vi "X_MN_4352.vi"(4 "u":dbl format="%#_13g") -> (1 "y":dbl)   [LabVIEW 2015]
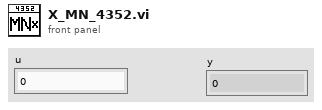
[diagram p1: front panel]
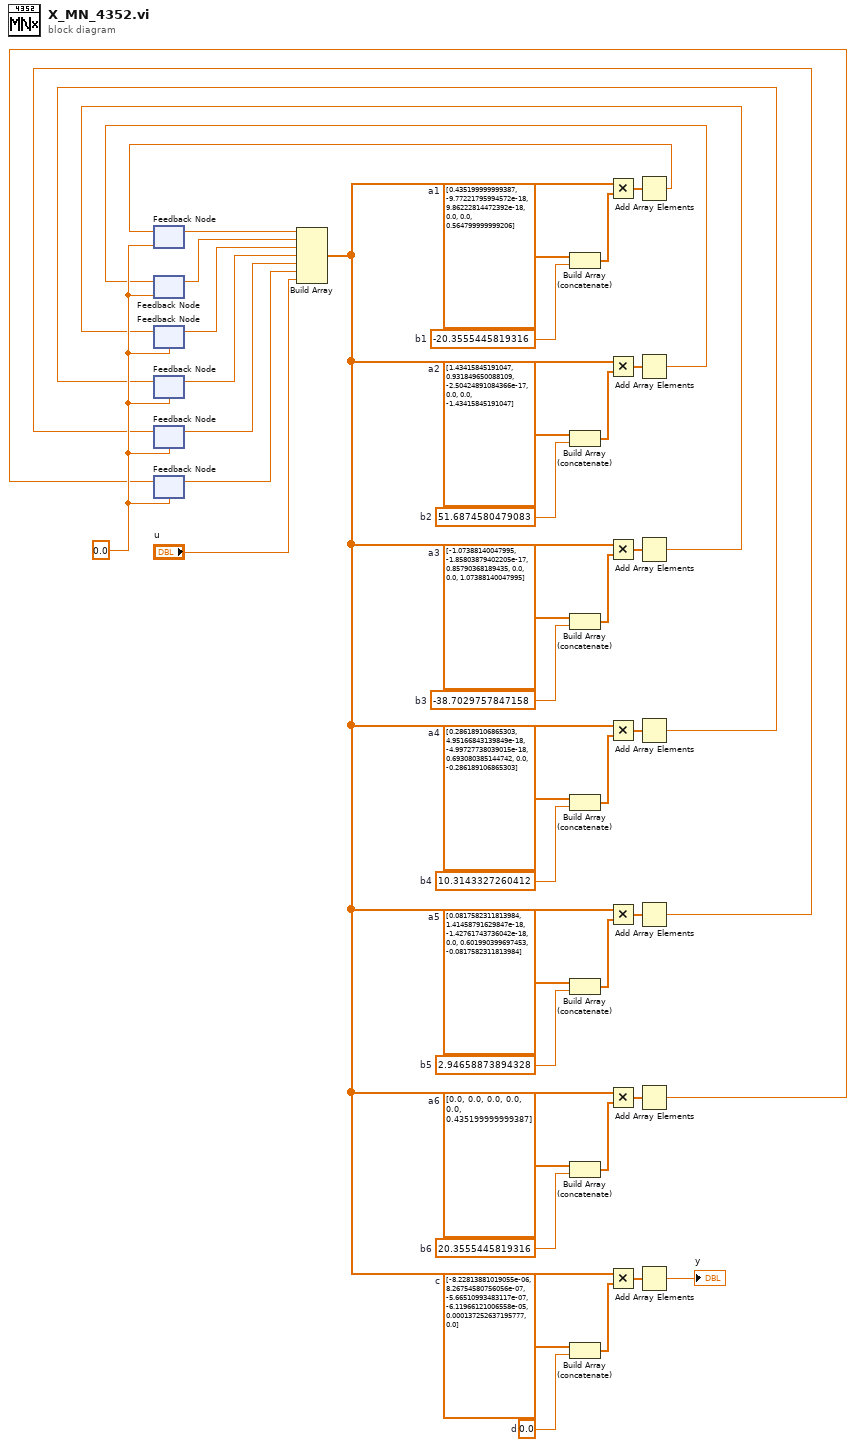
[diagram p0: block diagram]
diagram:
  w3 = 0.0  # d
  w2 = dbl[] [-8.22813881019055e-06, 8.26754580756056e-07, -5.66510993483117e-07, -6.11966121006558e-05, 0.000137252637195777, 0.0]  # c
  w5 = 20.3555445819316  # b6
  w6 = dbl[] [0.0, 0.0, 0.0, 0.0, 0.0, 0.435199999999387]  # a6
  w9 = 2.94658873894328  # b5
  w8 = dbl[] [0.0817582311813984, 1.41458791629847e-18, -1.42761743736042e-18, 0.0, 0.601990399697453, -0.0817582311813984]  # a5
  w11 = 10.3143327260412  # b4
  w12 = dbl[] [0.286189106865303, 4.95166843139849e-18, -4.99727738039015e-18, 0.693080385144742, 0.0, -0.286189106865303]  # a4
  w14 = -38.7029757847158  # b3
  w15 = dbl[] [-1.07388140047995, -1.85803879402205e-17, 0.85790368189435, 0.0, 0.0, 1.07388140047995]  # a3
  w18 = 51.6874580479083  # b2
  w17 = dbl[] [1.43415845191047, 0.931849650088109, -2.50424891084366e-17, 0.0, 0.0, -1.43415845191047]  # a2
  w20 = -20.3555445819316  # b1
  w21 = dbl[] [0.435199999999387, -9.77221795994572e-18, 9.86222814472392e-18, 0.0, 0.0, 0.564799999999206]  # a1
  w43 = 0.0
  n1 = feedback #1(w43) -> (w44:dbl)
  n2 = feedback #2(w43) -> (w42:dbl)
  n3 = feedback #3(w43) -> (w41:dbl)
  n4 = feedback #4(w43) -> (w40:dbl)
  n5 = feedback #5(w43) -> (w39:dbl)
  n6 = feedback #6(w43) -> (w38:dbl)
  n7 = Build Array(w44, w42, w41, w40, w39, w38, "u") -> (w33:dbl[])
  n8 = Build Array (concatenate)(w21, w20) -> (w19:dbl[])
  n9 = Build Array (concatenate)(w17, w18) -> (w16:dbl[])
  n10 = Build Array (concatenate)(w15, w14) -> (w13:dbl[])
  n11 = Build Array (concatenate)(w12, w11) -> (w10:dbl[])
  n12 = Build Array (concatenate)(w8, w9) -> (w7:dbl[])
  n13 = Build Array (concatenate)(w6, w5) -> (w4:dbl[])
  n14 = Build Array (concatenate)(w2, w3) -> (w1:dbl[])
  n15 = Multiply(x=w33, y=w19) -> (x*y=w35:dbl[])
  n16 = Multiply(x=w33, y=w16) -> (x*y=w32:dbl[])
  n17 = Multiply(x=w33, y=w13) -> (x*y=w31:dbl[])
  n18 = Multiply(x=w33, y=w10) -> (x*y=w30:dbl[])
  n19 = Multiply(x=w33, y=w7) -> (x*y=w29:dbl[])
  n20 = Multiply(x=w33, y=w4) -> (x*y=w28:dbl[])
  n21 = Multiply(x=w33, y=w1) -> (x*y=w37:dbl[])
  n22 = Add Array Elements(numeric array=w35) -> (sum=w27:dbl)
  n23 = feedback-in #1(w27) -> ()
  n24 = Add Array Elements(numeric array=w32) -> (sum=w26:dbl)
  n25 = feedback-in #2(w26) -> ()
  n26 = Add Array Elements(numeric array=w31) -> (sum=w25:dbl)
  n27 = feedback-in #3(w25) -> ()
  n28 = Add Array Elements(numeric array=w30) -> (sum=w24:dbl)
  n29 = feedback-in #4(w24) -> ()
  n30 = Add Array Elements(numeric array=w29) -> (sum=w23:dbl)
  n31 = feedback-in #5(w23) -> ()
  n32 = Add Array Elements(numeric array=w28) -> (sum=w22:dbl)
  n33 = feedback-in #6(w22) -> ()
  n34 = Add Array Elements(numeric array=w37) -> (sum=→"y":dbl)
